vi "chartsheet set header lv.vi"(8 "error in (no error)":errorcluster, 10 "header":string, 11 "chartsheet":u32) -> (0 "error out":errorcluster, 3 "function return":u32(ring))   [LabVIEW 8.6]
doc: "lxw_error chartsheet_set_header_lv(lxw_chartsheet chartsheet, const char *header);"
uses:
  pending_lvxlsxwriter/xlsxwriter.dll
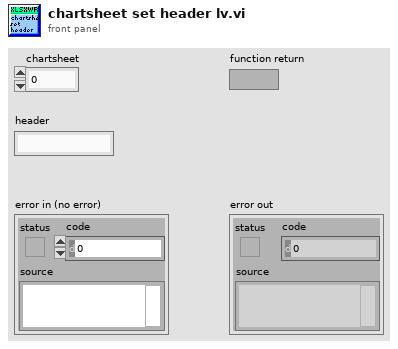
[diagram p1: front panel]
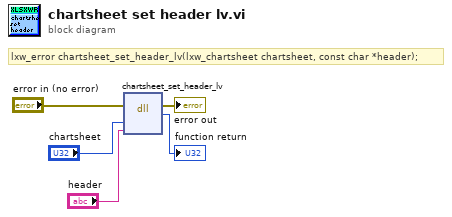
[diagram p0: block diagram]
diagram:
  # "lxw_error chartsheet_set_header_lv(lxw_chartsheet chartsheet, const char *header);"
  n1 = dll-call lib="C:/Users/WDAGUtilityAccount/Desktop/pending_lvxlsxwriter/xlsxwriter.*" fn="chartsheet_set_header_lv"(error in="error in (no error)", "chartsheet"="chartsheet", "header"="header") -> (error out=→"error out":errorcluster, →"function return":u32)  [unwired: 4 in, 1 out]
